vi "micro1 pvgen400.vi"(0 "FluxStrIn":string, 1 "Numin":i32, 5 "errin":errorcluster, 6 "testlabel":string, 7 "Data limit":dbl[](array[numeric]), 8 "tab ref":string[][](array[string]), 10 "ligne à traiter":string[](array[string])) -> (14 "result string":string, 15 "Numout":i32, 19 "errout":errorcluster)   [LabVIEW 2020]
uses:
  <vilib>/regexp/Match Regular Expression.xnode
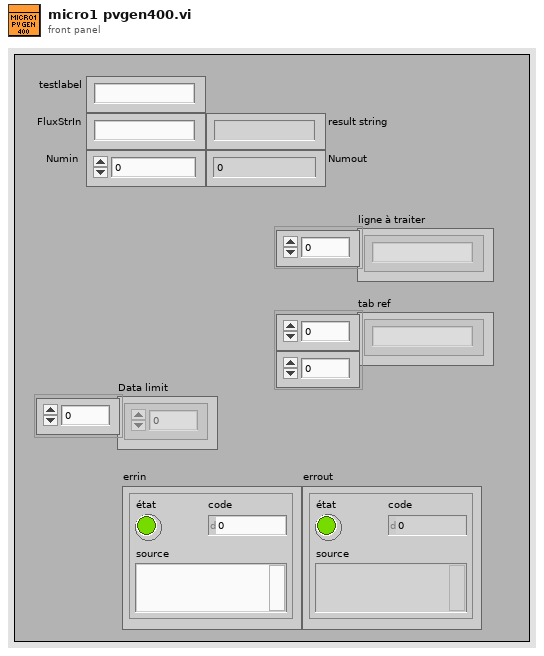
[diagram p1: front panel]
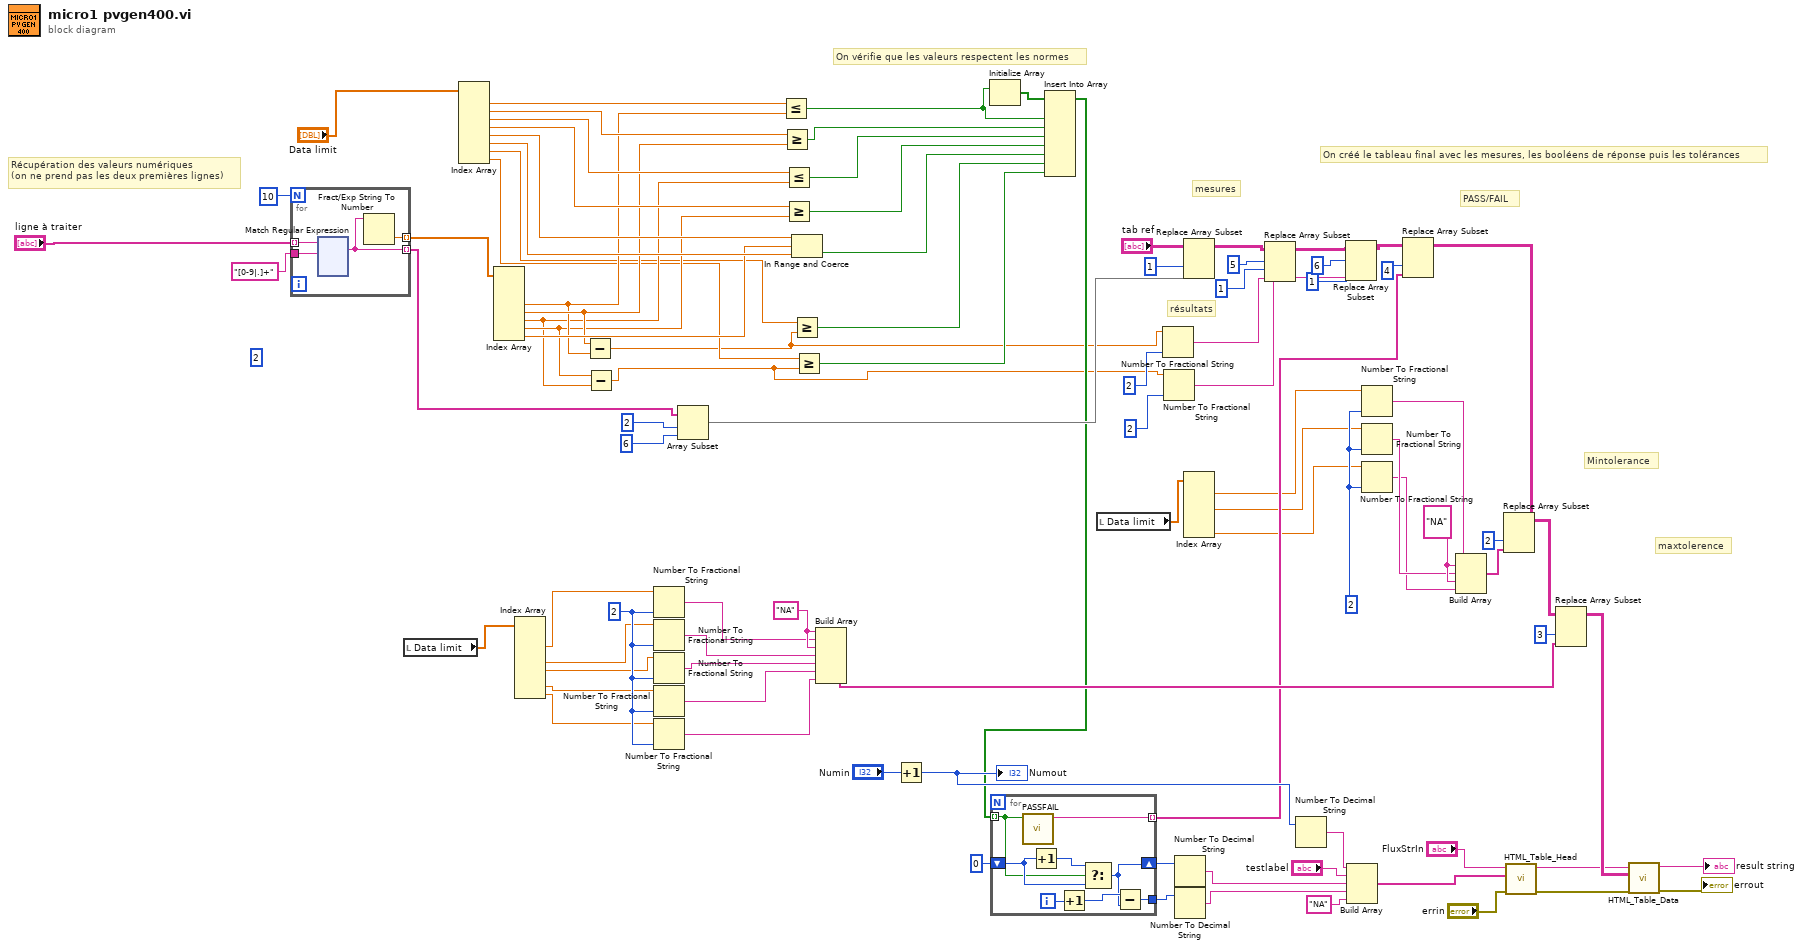
[diagram p0: block diagram]
diagram:
  w33 = "NA" ("element")
  w37 = "NA" ("element")
  (unwired) 2 ("indice")
  w47 = 2
  w57 = 2
  # "Récupération des valeurs numériques\n(on ne prend pas les deux premières lignes)"
  # "On créé le tableau final avec les mesures, les booléens de réponse puis les tolérances"
  # "On vérifie que les valeurs respectent les normes"
  # "maxtolerence"
  # "Mintolerance"
  # "mesures"
  # "PASS/FAIL"
  # "résultats"
  n1 = for {
    N: 10 -> [_]
    tunnel: "ligne à traiter" -> [w98] mode=indexing
    tunnel: "[0-9|.]+" ("expression régulière") -> [w97]
    tunnel: [w96] -> w54 mode=indexing
    tunnel: [w95] -> w53 mode=indexing
    n2 = xnode "Match Regular Expression"("input string"=w98, "regular expression"=w97) -> ("whole match"=w95:string)  [unwired: 4 in, 4 out]
    n3 = Fract/Exp String To Number(string=w95) -> (number=w96:dbl)  [unwired: 3 in, 1 out]
  }
  n4 = local read "Data limit"() -> (w55:dbl[])
  n5 = Index Array(array="Data limit") -> (element #1=w52:dbl, element #2=w51:dbl, element #3=w45:dbl, element #4=w44:dbl, element #5=w43:dbl, element #6=w42:dbl, element #7=w17:dbl, element #8=w16:dbl)  [unwired: 8 in]
  n6 = Index Array(array=w54) -> (element #3=w20:dbl, element #4=w21:dbl, element #5=w18:dbl, element #6=w19:dbl, element #7=w41:dbl)  [unwired: 7 in, 2 out]
  n7 = Index Array(array=w55) -> (element #2=w46:dbl, element #4=w32:dbl, element #5=w31:dbl, element #7=w30:dbl, element #8=w29:dbl)  [unwired: 8 in, 3 out]
  n8 = Subtract(x=w21, y=w20) -> (x-y=w11:dbl)
  n9 = Subtract(x=w19, y=w18) -> (x-y=w10:dbl)
  n10 = Number To Fractional String(number=w46, precision (6)=w47) -> (F-format string=w28:string)  [unwired: 2 in]
  n11 = Number To Fractional String(number=w32, precision (6)=w47) -> (F-format string=w27:string)  [unwired: 2 in]
  n12 = Number To Fractional String(number=w31, precision (6)=w47) -> (F-format string=w26:string)  [unwired: 2 in]
  n13 = Number To Fractional String(number=w30, precision (6)=w47) -> (F-format string=w24:string)  [unwired: 2 in]
  n14 = Number To Fractional String(number=w29, precision (6)=w47) -> (F-format string=w23:string)  [unwired: 2 in]
  n15 = Array Subset(array=w53, index=2 ("indice"), length=6 ("longueur")) -> (w63:string[])
  n16 = Less Or Equal?(x=w52, y=w20) -> (x <= y?=w22:bool)
  n17 = Greater Or Equal?(x=w51, y=w21) -> (x >= y?=w50:bool)
  n18 = Less Or Equal?(x=w45, y=w18) -> (x <= y?=w40:bool)
  n19 = Greater Or Equal?(x=w44, y=w19) -> (x >= y?=w39:bool)
  n20 = In Range and Coerce(upper limit=w43, x=w41, lower limit=w42) -> (In Range?=w38:bool)  [unwired: 1 out]
  n21 = Greater Or Equal?(x=w17, y=w11) -> (x >= y?=w15:bool)
  n22 = Greater Or Equal?(x=w16, y=w10) -> (x >= y?=w14:bool)
  n23 = Build Array(w33, w28, w33, w27, w26, w24, w23) -> (w94:string[])
  n24 = Increment(x="Numin") -> (x+1=w80:i32)
  "Numout" <- w80
  n25 = Initialize Array(w22) -> (w49:bool[])  [unwired: 1 in]
  n26 = Insert Into Array(array=w49, new element #1=w22, new element #2=w50, new element #3=w40, new element #4=w39, new element #5=w38, new element #6=w15, new element #7=w14) -> (w59:bool[])  [unwired: 1 in]
  n27 = for {
    tunnel: w59 -> [w214] mode=indexing
    tunnel: [w213] -> w60 mode=indexing
    shift-right: [w216] -> w82
    shift-left: 0 -> [w219]
    tunnel: [w215] -> w83
    i -> [w218]
    n28 = call "PASSFAIL.vi"("E"=w214) -> ("S"=w213:string)  [unwired: 10 in]
    n29 = Increment(x=w219) -> (x+1=w220:i32)
    n30 = Increment(x=w218) -> (x+1=w217:i32)
    n31 = Select(t=w220, s=w214, f=w219) -> (s? t:f=w216:i32)
    n32 = Subtract(x=w217, y=w216) -> (x-y=w215:i32)
  }
  n33 = local read "Data limit"() -> (w56:dbl[])
  n34 = Number To Fractional String(number=w11, precision (6)=i16 2) -> (F-format string=w4:string)  [unwired: 2 in]
  n35 = Number To Fractional String(number=w10, precision (6)=i16 2) -> (F-format string=w1:string)  [unwired: 2 in]
  n36 = Number To Decimal String(number=w82) -> (decimal integer string=w84:string)  [unwired: 1 in]
  n37 = Number To Decimal String(number=w83) -> (decimal integer string=w85:string)  [unwired: 1 in]
  n38 = Replace Array Subset(array="tab ref", new element=w63, index (col)=1 ("indice désactivé (col)")) -> (w8:string[][])  [unwired: 1 in]
  n39 = Index Array(array=w56) -> (element #1=w48:dbl, element #3=w34:dbl, element #6=w36:dbl)  [unwired: 6 in, 3 out]
  n40 = Replace Array Subset(array=w8, new element=w4, index (row)=5 ("disabled index (row)"), index (col)=1 ("disabled index (col)")) -> (w6:string[][])
  n41 = Number To Decimal String(number=w80) -> (decimal integer string=w68:string)  [unwired: 1 in]
  n42 = Replace Array Subset(array=w6, new element=w1, index (row)=6 ("disabled index (row)"), index (col)=1 ("disabled index (col)")) -> (w5:string[][])
  n43 = Build Array(w68, "testlabel", w84, w85, "NA" ("élément")) -> (w71:string[])
  n44 = Number To Fractional String(number=w48, precision (6)=w57) -> (F-format string=w58:string)  [unwired: 2 in]
  n45 = Number To Fractional String(number=w34, precision (6)=w57) -> (F-format string=w35:string)  [unwired: 2 in]
  n46 = Number To Fractional String(number=w36, precision (6)=w57) -> (F-format string=w25:string)  [unwired: 2 in]
  n47 = Replace Array Subset(array=w5, new element=w60, index (col)=4 ("indice désactivé (col)")) -> (w88:string[][])  [unwired: 1 in]
  n48 = Build Array(w58, w37, w35, w37, w25) -> (w93:string[])
  n49 = Replace Array Subset(array=w88, new element=w93, index (col)=2 ("indice désactivé (col)")) -> (w90:string[][])  [unwired: 1 in]
  n50 = call "HTML_Table_Head.vi"("entrée d'erreur (pas d'erreur)"="errin", "Tableau"=w71, "chaîne en entrée"="FluxStrIn") -> ("sortie d'erreur"=w70:errorcluster, "result string"=w69:string)  [unwired: 7 in]
  n51 = Replace Array Subset(array=w90, new element=w94, index (col)=3 ("indice désactivé (col)")) -> (w89:string[][])  [unwired: 1 in]
  n52 = call "HTML_Table_Data.vi"("entrée d'erreur (pas d'erreur)"=w70, "Tableau"=w89, "chaîne en entrée"=w69) -> ("sortie d'erreur"=→"errout":errorcluster, "result string"=→"result string":string)  [unwired: 7 in]
